vi "Get Active Plugins.vi"(8 "error in (no error)":errorcluster, 11 "Configuration Manager In":refnum<class "Configuration Manager.lvclass">) -> (0 "error out":errorcluster, 2 "Plugins":string[](array[string]), 3 "Configuration Manager Out":refnum<class "Configuration Manager.lvclass">)   [LabVIEW 2020, in "Configuration Manager.lvclass"]
uses:
  Configuration Manager.lvclass
  Configuration Manager.lvclass/Configuration Manager.ctl
  <vilib>/Utility/config.llb/Read Key (Boolean).vi
  <vilib>/Utility/config.llb/NI_LVConfig.lvlib
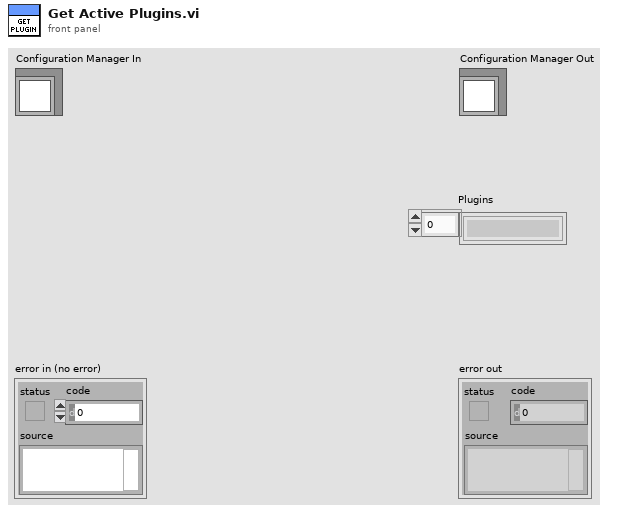
[diagram p1: front panel]
types:
  T1 = typedef "NI_LVConfig.lvlib/Config Data RefNum.ctl" = refnum<k1>
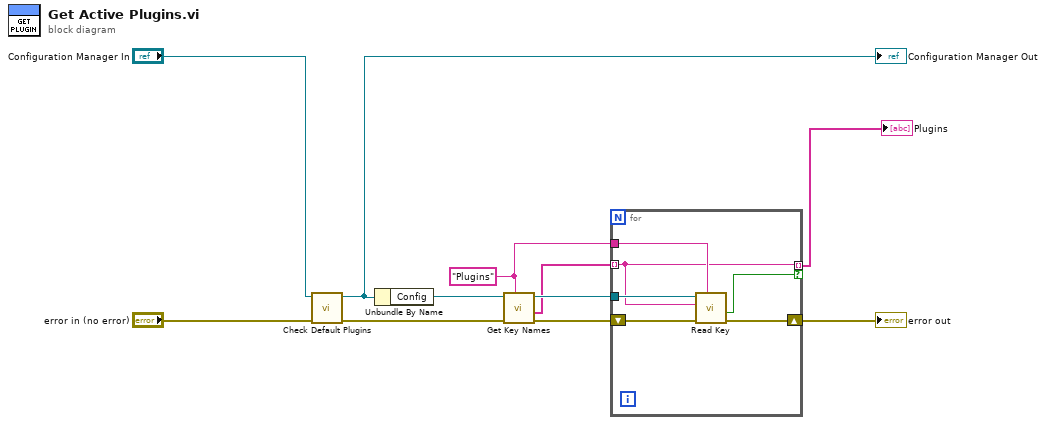
[diagram p0: block diagram]
diagram:
  w5 = "Plugins" ("section")
  n1 = call "Check Default Plugins.vi"("error in (no error)"="error in (no error)", "Configuration Manager in"="Configuration Manager In") -> ("error out"=w3:errorcluster, "Configuration Manager out"=w1:refnum<class "Configuration Manager.lvclass">)  [unwired: 8 in]
  "Configuration Manager Out" <- w1
  n2 = Unbundle By Name(w1) -> ("Config"=w9:T1)
  n3 = call <vilib>:"Get Key Names.vi"("section"=w5, "error in (no error)"=w3, "refnum"=w9) -> ("error out"=w10:errorcluster, "key names"=w6:string[], "refnum out"=w7:T1)  [unwired: 5 in, 1 out]
  n4 = for {
    shift-right: [w16] -> w8
    shift-left: w10 -> [w17]
    tunnel: w7 -> [w15]
    tunnel: w6 -> [w13] mode=indexing
    tunnel: w5 -> [w14]
    tunnel: [w13] -> w4 mode=indexing if=w12
    n5 = call-poly <vilib>:"Read Key.vi"("section"=w14, "error in (no error)"=w17, "key"=w13, "refnum"=w15) -> ("error out"=w16:errorcluster, "value"=w12:bool)  [unwired: 4 in, 2 out]
  }
  "error out" <- w8
  "Plugins" <- w4
